vi "Check for 'Wait' Errors.vi"(8 "error in (no error)":errorcluster, 10 "return code":dbl) -> (0 "error out":errorcluster, 2 "return code out":dbl)   [LabVIEW 2009, in "HighFinesse WS5.lvlib"]
doc: "Takes the result of a WaitForWLMEvent call to the wavelength meter and checks for errors."
uses:
  HighFinesse WS5.lvlib
  <vilib>/Utility/error.llb/DialogType.ctl
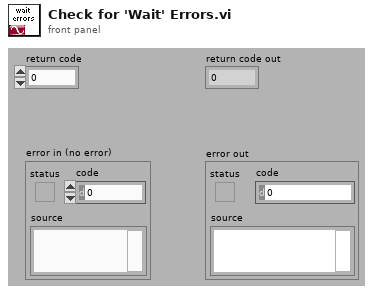
[diagram p1: front panel]
types:
  T1 = typedef "DialogType.ctl" = u16
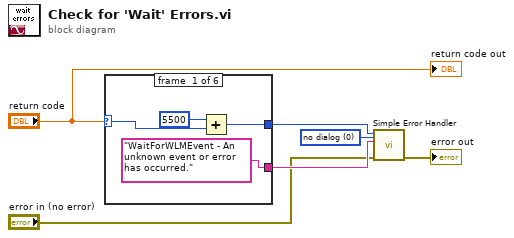
[diagram p0: block diagram]
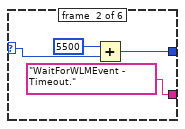
[diagram p2: hidden frame]
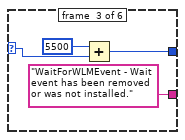
[diagram p3: hidden frame]
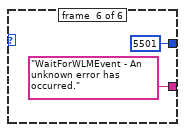
[diagram p6: hidden frame]
diagram:
  w6 = T1 0 items=["no dialog", "OK message", "continue or stop message", "OK message + warnings", "continue/stop + warnings"] ("type of dialog (OK msg:1)")
  n1 = case shown="Default" "return code" {
    selector: "return code" -> [w8 w12 w17 _ _ _]
    tunnel: ["WaitForWLMEvent - An unknown event or error has occurred." ("error source (\" \")") "WaitForWLMEvent - Timeout." ("error source (\" \")") "WaitForWLMEvent - Wait event has been removed or was not installed." ("error source (\" \")") _ _ "WaitForWLMEvent - An unknown error has occurred." ("error source (\" \")")] -> w5
    tunnel: [w7 w11 w15 _ _ 5501 ("x")] -> w2
    frame #0 {
      n2 = Add(x=5500, y=w8) -> (x+y=w7:i32)
    }
    frame #1 {
      n3 = Add(x=5500, y=w12) -> (x+y=w11:i32)
    }
    frame #2 {
      n4 = Add(x=5500, y=w17) -> (x+y=w15:i32)
    }
    frame #3 {
    }
    frame #4 {
    }
    frame #5 {
    }
  }
  n5 = call <vilib>:"Simple Error Handler.vi"("error code (no error:0)"=w2, "error source (\" \")"=w5, "type of dialog (OK msg:1)"=w6, "error in (no error)"="error in (no error)") -> ("error out"=→"error out":errorcluster)  [unwired: 5 out]
  "return code out" <- "return code"
